vi "Main.vi"() -> ()   [LabVIEW 2019]
uses:
  States Enum.ctl
  Data Cluster.ctl
  <vilib>/express/express analysis/Spectral/Block/exnSpectralBlock spectral measurements RMS poly.vi
  <vilib>/express/express analysis/Spectral/Block/exnSpectralBlock spectral measurements RMS DDT.vi
  <vilib>/express/express analysis/Spectral/XNode/ExpressSpectralMeasurementsBlockNode.xnode
panel:
  out "Empty Channel":dynamicdata(graph)
  out "FFT 4":dynamicdata(graph)
  out "PZT Sensor":dynamicdata(graph)
  out "FFT 3":dynamicdata(graph)
  in  "Stop":bool
  in  "file path":path=path "C:/Users/lycan/OneDrive - The Ohio State University/Academics/Softwares/Labview/Frequency Analyzer/Frequency Analyzer Folder for LV19/OneDrive - The Ohio State University/Academics/Softwares/Labview/Frequency Analyzer/Test.xlsx.tdms"
  out "Drive Frequency (Hz)":dbl
  in  "Step Interval (ms)":dbl=100.0 min=0.2 max=5000000.0 step=0.1 format="%#.2p"
  in  "Step (Hz)":dbl=100.0 min=0.2 max=5000000.0 step=0.1 format="%#.2p"
  in  "Stop Frequency (Hz)":dbl=100.0 min=0.2 max=5000000.0 step=0.1 format="%#.2p"
  in  "Start Frequency(Hz)":dbl=100.0 min=0.2 max=5000000.0 step=0.1 format="%#.2p"
  in  "Amplitude (Vpp)":dbl=1.0 min=0.0 max=10.0 step=0.01 format="%#.2p"
  in  "Signal Route":u16(ring)=1 items=["Prototyping board", "FGEN BNC", "AO 0", "AO 1"]
  in  "Type":u16(ring) items=["Sine", "Triangle", "Square"]
  out "Microphone":dynamicdata(graph)
  out "FFT 2":dynamicdata(graph)
  out "FFT":dynamicdata(graph)
  out "PZT Actuator":dynamicdata(graph)
  # "Function Generator and Signal Analyzer"
  # "Error Message:"
  # "V 1.0"
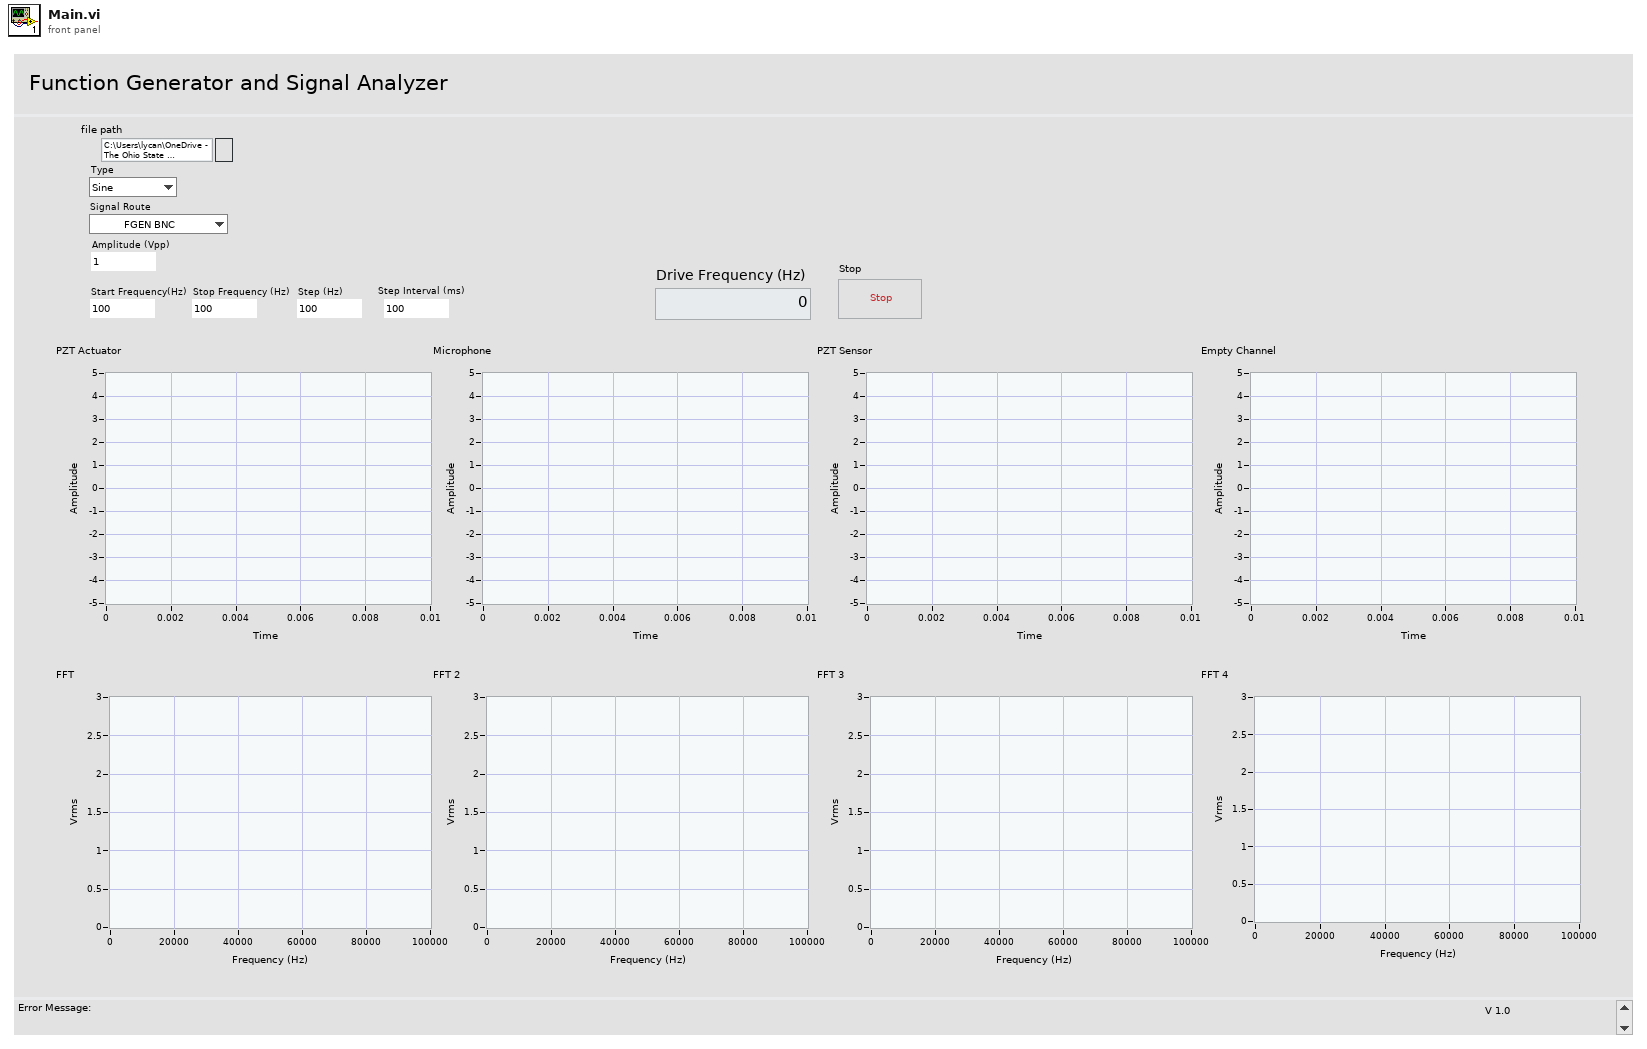
[diagram p1: front panel]
types:
  T1 = enum16{"open", "open or create", "create or replace", "create", "open (read-only)"}
  T2 = typedef "Data Cluster.ctl" = cluster{"Scope 1 Data":dbl[][], "Drive Frequency":dbl, "Scope 2 Data":dbl[][], "Scope 3 Data":dbl[][], "Scope 4 Data":dbl[][]}
  T3 = typedef "States Enum.ctl" = enum16{"Scope3", "Scope4", "Function Generator", "Scope1", "Scope2", "Stepping"}
  T4 = cluster{"averaging mode":u16, "weighting mode":u16, "number of averages":u32}
  T5 = cluster{"dB On (F)":bool, "unwrap phase (F)":bool, "convert to degree (F)":bool}
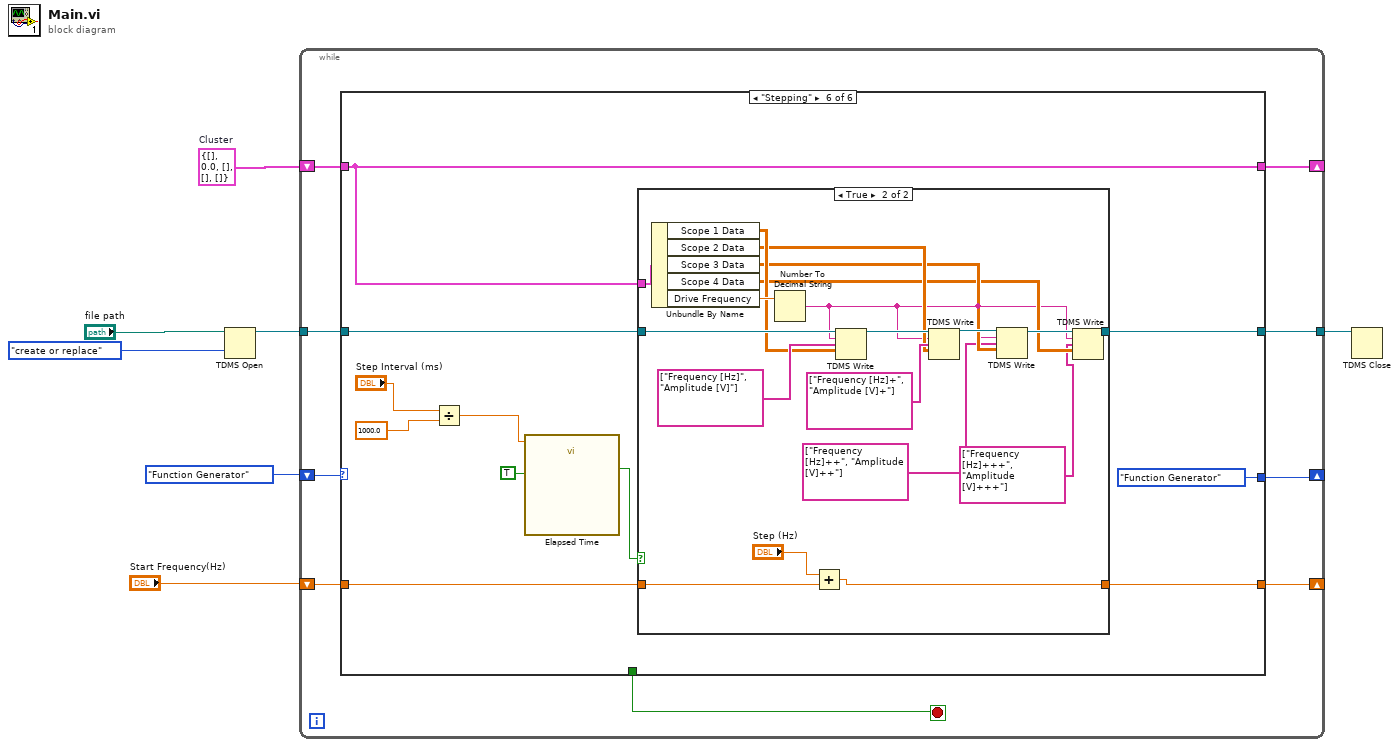
[diagram p0: block diagram]
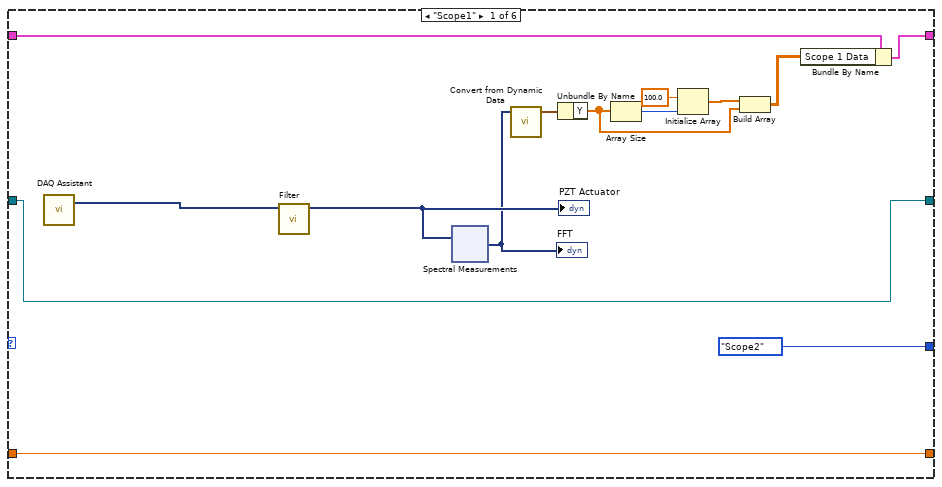
[diagram p2: hidden frame]
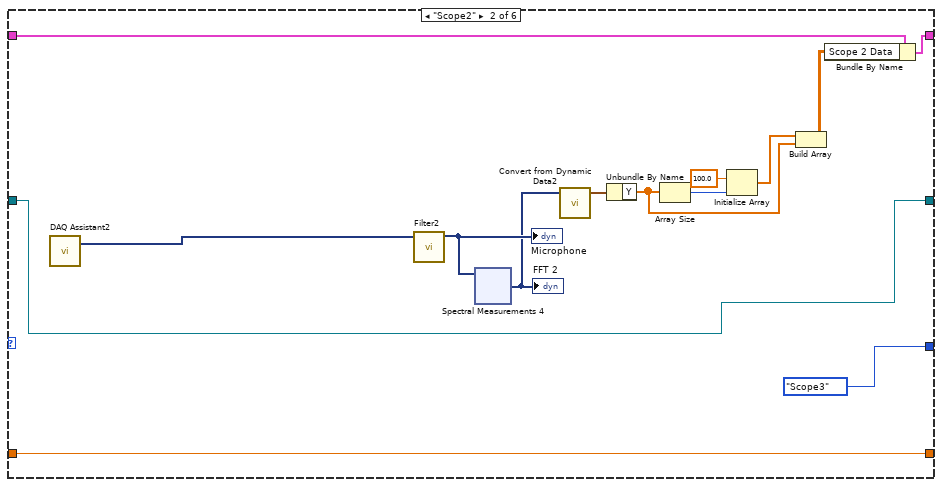
[diagram p3: hidden frame]
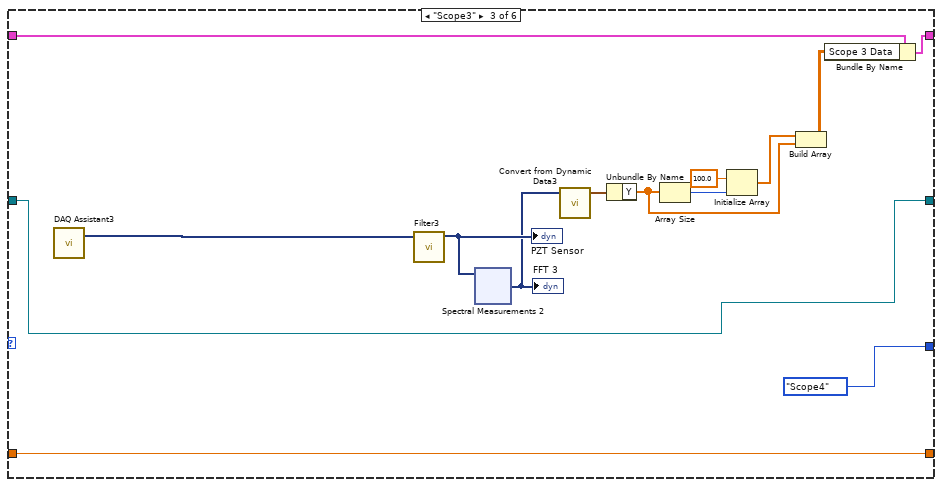
[diagram p4: hidden frame]
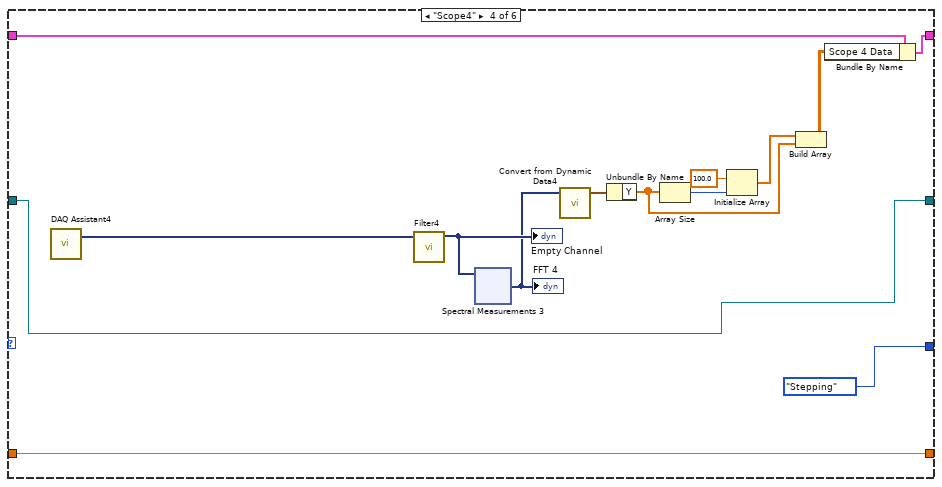
[diagram p5: hidden frame]
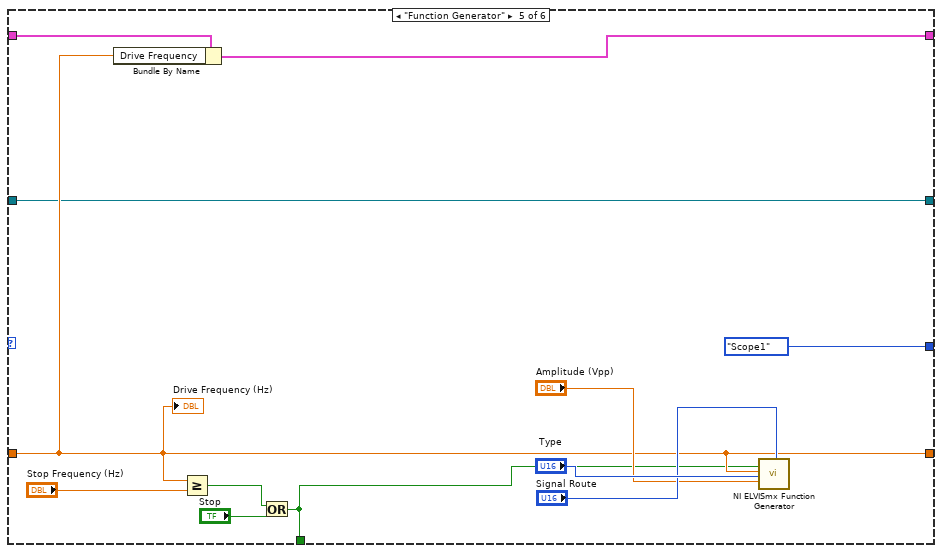
[diagram p6: hidden frame]
diagram:
  w5 = T2 {"Scope 1 Data"=[], "Drive Frequency"=0.0, "Scope 2 Data"=[], "Scope 3 Data"=[], "Scope 4 Data"=[]}  # Cluster
  n1 = TDMS Open(10:T1."create or replace" ("operation (0:open)"), 11:"file path") -> (3:w4:refnum<k34>)  [unwired: 5 in, 1 out]
  n2 = while {
    shift-right: [w16] -> _
    shift-left: States_Enum."Function Generator" ("Enum") -> [w15]
    shift-right: [w13] -> _
    shift-left: "Start Frequency(Hz)" -> [w14]
    shift-right: [w10] -> _
    shift-left: w5 -> [w11]
    tunnel: w4 -> [w9]
    tunnel: [w8] -> w3
    stop <- w12 stop-if-true
    n3 = case shown="\"Stepping\"" w15 {
      tunnel: [States_Enum."Scope2" ("Enum") States_Enum."Scope3" ("Enum") States_Enum."Scope4" ("Enum") States_Enum."Stepping" ("Enum") States_Enum."Scope1" ("Enum") States_Enum."Function Generator" ("Enum")] -> w16
      tunnel: w14 -> [w28 w52 w77 w102 w122 w137]
      tunnel: [w28 w52 w77 w102 w122 w132] -> w13
      tunnel: [_ _ _ _ w117 _] -> w12
      tunnel: w11 -> [w22 w45 w70 w95 w123 w129]
      tunnel: [w21 w42 w67 w92 w121 w129] -> w10
      tunnel: w9 -> [w19 w43 w68 w93 w120 w131]
      tunnel: [w19 w43 w68 w93 w120 w130] -> w8
      frame "Scope1" {
        n4 = call "DAQ Assistant"() -> ("data"=w30:dynamicdata)  [unwired: 17 in, 2 out]
        n5 = call "Filter"("Signal"=w30) -> ("Filtered Signal"=w18:dynamicdata)  [unwired: 9 in, 1 out]
        "PZT Actuator" <- w18
        n6 = xnode "Spectral Measurements"("Signals"=w18) -> ("FFT - (RMS)"=w17:dynamicdata)  [unwired: 2 in, 3 out]
        "FFT" <- w17
        n7 = call "Convert from Dynamic Data"("Dynamic Data Type"=w17) -> ("Waveform"=w27:waveform(dbl))  [unwired: 3 in]
        n8 = Unbundle By Name(w27) -> ("Y"=w23:dbl[])
        n9 = Array Size(array=w23) -> (size(s)=w26:i32)
        n10 = Initialize Array(100.0 ("element"), w26) -> (w24:dbl[])
        n11 = Build Array(w24, w23) -> (w20:dbl[][])
        n12 = Bundle By Name(cluster=w22, "Scope 1 Data"=w20) -> (w21:T2)
      }
      frame "Scope2" {
        n13 = call "DAQ Assistant2"() -> ("data"=w54:dynamicdata)  [unwired: 17 in, 2 out]
        n14 = call "Filter2"("Signal"=w54) -> ("Filtered Signal"=w55:dynamicdata)  [unwired: 9 in, 1 out]
        "Microphone" <- w55
        n15 = xnode "Spectral Measurements 4"("Signals"=w55) -> ("FFT - (RMS)"=w46:dynamicdata)  [unwired: 2 in, 3 out]
        "FFT 2" <- w46
        n16 = call "Convert from Dynamic Data2"("Dynamic Data Type"=w46) -> ("Waveform"=w51:waveform(dbl))  [unwired: 3 in]
        n17 = Unbundle By Name(w51) -> ("Y"=w47:dbl[])
        n18 = Array Size(array=w47) -> (size(s)=w50:i32)
        n19 = Initialize Array(100.0 ("element"), w50) -> (w48:dbl[])
        n20 = Build Array(w48, w47) -> (w44:dbl[][])
        n21 = Bundle By Name(cluster=w45, "Scope 2 Data"=w44) -> (w42:T2)
      }
      frame "Scope3" {
        n22 = call "DAQ Assistant3"() -> ("data"=w79:dynamicdata)  [unwired: 17 in, 2 out]
        n23 = call "Filter3"("Signal"=w79) -> ("Filtered Signal"=w80:dynamicdata)  [unwired: 9 in, 1 out]
        "PZT Sensor" <- w80
        n24 = xnode "Spectral Measurements 2"("Signals"=w80) -> ("FFT - (RMS)"=w71:dynamicdata)  [unwired: 2 in, 3 out]
        "FFT 3" <- w71
        n25 = call "Convert from Dynamic Data3"("Dynamic Data Type"=w71) -> ("Waveform"=w76:waveform(dbl))  [unwired: 3 in]
        n26 = Unbundle By Name(w76) -> ("Y"=w72:dbl[])
        n27 = Array Size(array=w72) -> (size(s)=w75:i32)
        n28 = Initialize Array(100.0 ("element"), w75) -> (w73:dbl[])
        n29 = Build Array(w73, w72) -> (w69:dbl[][])
        n30 = Bundle By Name(cluster=w70, "Scope 3 Data"=w69) -> (w67:T2)
      }
      frame "Scope4" {
        n31 = call "DAQ Assistant4"() -> ("data"=w104:dynamicdata)  [unwired: 17 in, 2 out]
        n32 = call "Filter4"("Signal"=w104) -> ("Filtered Signal"=w105:dynamicdata)  [unwired: 9 in, 1 out]
        "Empty Channel" <- w105
        n33 = xnode "Spectral Measurements 3"("Signals"=w105) -> ("FFT - (RMS)"=w96:dynamicdata)  [unwired: 2 in, 3 out]
        "FFT 4" <- w96
        n34 = call "Convert from Dynamic Data4"("Dynamic Data Type"=w96) -> ("Waveform"=w101:waveform(dbl))  [unwired: 3 in]
        n35 = Unbundle By Name(w101) -> ("Y"=w97:dbl[])
        n36 = Array Size(array=w97) -> (size(s)=w100:i32)
        n37 = Initialize Array(100.0 ("element"), w100) -> (w98:dbl[])
        n38 = Build Array(w98, w97) -> (w94:dbl[][])
        n39 = Bundle By Name(cluster=w95, "Scope 4 Data"=w94) -> (w92:T2)
      }
      frame "Function Generator" {
        n40 = Bundle By Name(cluster=w123, "Drive Frequency"=w122) -> (w121:T2)
        n41 = Greater Or Equal?(x=w122, y="Stop Frequency (Hz)") -> (x >= y?=w119:bool)
        n42 = Or(x=w119, y="Stop") -> (x .or. y?=w117:bool)
        n43 = call "NI ELVISmx Function Generator"("Stop"=w117, "Frequency (Hz)"=w122, "Amplitude (Vpp)"="Amplitude (Vpp)", "Type"="Type", "Signal Route"="Signal Route") -> ()  [unwired: 13 in, 2 out]
        "Drive Frequency (Hz)" <- w122
      }
      frame "Stepping" {
        n44 = Divide(x="Step Interval (ms)", y=1000.0) -> (x/y=w134:dbl)
        n45 = call "Elapsed Time"("Time Target (s)"=w134, "Auto Reset"=TRUE) -> ("Time has Elapsed"=w138:bool)  [unwired: 10 in, 7 out]
        n46 = case shown="True" w138 {
          tunnel: w137 -> [w141 w159]
          tunnel: [w141 w158] -> w132
          tunnel: w129 -> [_ w156]
          tunnel: w131 -> [w140 w153]
          tunnel: [w140 w151] -> w130
          frame False {
          }
          frame True {
            n47 = Unbundle By Name(w156) -> ("Scope 1 Data"=w148:dbl[][], "Scope 2 Data"=w147:dbl[][], "Scope 3 Data"=w146:dbl[][], "Scope 4 Data"=w145:dbl[][], "Drive Frequency"=w155:dbl)
            n48 = Number To Decimal String(number=w155) -> (decimal integer string=w142:string)  [unwired: 1 in]
            n49 = Add(x="Step (Hz)", y=w159) -> (x+y=w158:dbl)
            n50 = TDMS Write(0:w153, 5:w142, 7:string[] ["Frequency [Hz]", "Amplitude [V]"] ("channel name(s) in (Untitled)"), 9:w148) -> (4:w157:refnum<k34>)  [unwired: 2 in, 3 out]
            n51 = TDMS Write(0:w157, 5:w142, 7:string[] ["Frequency [Hz]+", "Amplitude [V]+"] ("channel name(s) in (Untitled)"), 9:w147) -> (4:w149:refnum<k34>)  [unwired: 2 in, 3 out]
            n52 = TDMS Write(0:w149, 5:w142, 7:string[] ["Frequency [Hz]++", "Amplitude [V]++"] ("channel name(s) in (Untitled)"), 9:w146) -> (4:w150:refnum<k34>)  [unwired: 2 in, 3 out]
            n53 = TDMS Write(0:w150, 5:w142, 7:string[] ["Frequency [Hz]+++", "Amplitude [V]+++"] ("channel name(s) in (Untitled)"), 9:w145) -> (4:w151:refnum<k34>)  [unwired: 2 in, 3 out]
          }
        }
      }
    }
  }
  n54 = TDMS Close(11:w3) -> ()  [unwired: 1 in, 2 out]
